vi "Main_Target.vi"() -> ()   [LabVIEW 2018]
uses:
  Tasks_RT.ctl
  ActionCluster.ctl
  Instructions_RT.ctl
  ParameterSubCluster.ctl
panel:
  out "Chart 2":i16(graph)
  out "Chart":u16(graph)
  out "Inbit line":string="6509/port0/line1"
  in  "Action cluster":T1={"Macro Instructions"=[{"Duration (s)"=0.1, "Steps"=1, "Changes"=[FALSE, TRUE, FALSE], "Triggers"=[], "RAW cmds 2D"=[[0, 0, 0, 0, 0, 0, 0, 0], [0, 0, 0, 0, 0, 0, 0, 0], [0, 0, 0, 0, 0, 0, 0, 0], [0, 0, 0, 0, 0, 0, 0, 0], [0, 0, 0, 0, 0, 0, 0, 0], [0, 0, 0, 0, 0, 0, 0, 0], [0, 0, 0, 0, 0, 0, 0, 0], [0, 0, 0, 0, 0, 0, 0, 0], [0, 0, 0, 0, 0, 0, 0, 0], [0, 0, 0, 0, 0, 0, 0, 0], [0, 0, 0, 0, 0, 0, 0, 0], [0, 0, 0, 0, 0, 0, 0, 0], [0, 0, 0, 0, 0, 0, 0, 0], [0, 0, 0, 0, 0, 0, 0, 0], [0, 0, 0, 0, 0, 0, 0, 0], [0, 0, 0, 0, 0, 0, 0, 0], [0, 0, 0, 0, 0, 0, 0, 0], [0, 0, 0, 0, 0, 0, 0, 0], [0, 0, 0, 0, 0, 0, 0, 0], [0, 0, 0, 0, 0, 0, 0, 0], [0, 0, 0, 0, 0, 0, 0, 0], [0, 0, 0, 0, 0, 0, 0, 0], [0, 0, 0, 0, 0, 0, 0, 0], [0, 0, 0, 0, 0, 0, 0, 0], [0, 0, 0, 0, 0, 0, 0, 0], [0, 0, 0, 0, 0, 0, 0, 0], [0, 0, 0, 0, 0, 0, 0, 0], [0, 0, 0, 0, 0, 0, 0, 0], [0, 0, 0, 0, 0, 0, 0, 0], [0, 0, 0, 0, 0, 0, 0, 0], [0, 0, 0, 0, 0, 0, 0, 0], [0, 0, 0, 0, 0, 0, 0, 0], [0, 0, 0, 0, 0, 0, 0, 0], [0, 0, 0, 0, 0, 0, 0, 0], [0, 0, 0, 0, 0, 0, 0, 0], [0, 0, 0, 0, 0, 0, 0, 0], [0, 0, 0, 0, 0, 0, 0, 0], [0, 0, 0, 0, 0, 0, 0, 0], [0, 0, 0, 0, 0, 0, 0, 0], [0, 0, 0, 0, 0, 0, 0, 0], [0, 0, 0, 0, 0, 0, 0, 0], [0, 0, 0, 0, 0, 0, 0, 0], [0, 0, 0, 0, 0, 0, 0, 0], [0, 0, 0, 0, 0, 0, 0, 0], [0, 0, 0, 0, 0, 0, 0, 0], [0, 0, 0, 0, 0, 0, 0, 0], [0, 0, 0, 0, 0, 0, 0, 0], [0, 0, 0, 0, 0, 0, 0, 0], [0, 0, 0, 0, 0, 0, 0, 0], [0, 0, 0, 0, 0, 0, 0, 0], [0, 0, 0, 0, 0, 0, 0, 0], [0, 0, 0, 0, 0, 0, 0, 0], [0, 0, 0, 0, 0, 0, 0, 0], [0, 0, 0, 0, 0, 0, 0, 0], [0, 0, 0, 0, 0, 0, 0, 0], [0, 0, 0, 0, 0, 0, 0, 0], [0, 0, 0, 0, 0, 0, 0, 0], [0, 0, 0, 0, 0, 0, 0, 0], [0, 0, 0, 0, 0, 0, 0, 0], [0, 0, 0, 0, 0, 0, 0, 0], [0, 0, 0, 0, 0, 0, 0, 0], [0, 0, 0, 0, 0, 0, 0, 0], [0, 0, 0, 0, 0, 0, 0, 0], [0, 0, 0, 0, 0, 0, 0, 0], [0, 0, 0, 0, 0, 0, 0, 0], [0, 0, 0, 0, 0, 0, 0, 0], [0, 0, 0, 0, 0, 0, 0, 0], [0, 0, 0, 0, 0, 0, 0, 0], [0, 0, 0, 0, 0, 0, 0, 0], [0, 0, 0, 0, 0, 0, 0, 0], [0, 0, 0, 0, 0, 0, 0, 0], [0, 0, 0, 0, 0, 0, 0, 0], [0, 0, 0, 0, 0, 0, 0, 0], [0, 0, 0, 0, 0, 0, 0, 0], [0, 0, 0, 0, 0, 0, 0, 0], [0, 0, 0, 0, 0, 0, 0, 0], [0, 0, 0, 0, 0, 0, 0, 0], [0, 0, 0, 0, 0, 0, 0, 0], [0, 0, 0, 0, 0, 0, 0, 0], [0, 0, 0, 0, 0, 0, 0, 0], [0, 0, 0, 0, 0, 0, 0, 0], [0, 0, 0, 0, 0, 0, 0, 0], [0, 0, 0, 0, 0, 0, 0, 0], [0, 0, 0, 0, 0, 0, 0, 0], [0, 0, 0, 0, 0, 0, 0, 0], [0, 0, 0, 0, 0, 0, 0, 0], [0, 0, 0, 0, 0, 0, 0, 0], [0, 0, 0, 0, 0, 0, 0, 0], [0, 0, 0, 0, 0, 0, 0, 0], [0, 0, 0, 0, 0, 0, 0, 0], [0, 0, 0, 0, 0, 0, 0, 0], [0, 0, 0, 0, 0, 0, 0, 0], [0, 0, 0, 0, 0, 0, 0, 0], [0, 0, 0, 0, 0, 0, 0, 0], [0, 0, 0, 0, 0, 0, 0, 0], [0, 0, 0, 0, 0, 0, 0, 0], [0, 0, 0, 0, 0, 0, 0, 0], [0, 0, 0, 0, 0, 0, 0, 0], [0, 0, 0, 0, 0, 0, 0, 0], [0, 0, 0, 0, 0, 0, 0, 0], [0, 0, 0, 0, 0, 0, 0, 0], [0, 0, 0, 0, 0, 0, 0, 0], [0, 0, 0, 0, 0, 0, 0, 0], [0, 0, 0, 0, 0, 0, 0, 0], [0, 0, 0, 0, 0, 0, 0, 0], [0, 0, 0, 0, 0, 0, 0, 0], [0, 0, 0, 0, 0, 0, 0, 0], [0, 0, 0, 0, 0, 0, 0, 0], [0, 0, 0, 0, 0, 0, 0, 0], [0, 0, 0, 0, 0, 0, 0, 0], [0, 0, 0, 0, 0, 0, 0, 0], [0, 0, 0, 0, 0, 0, 0, 0], [0, 0, 0, 0, 0, 0, 0, 0], [0, 0, 0, 0, 0, 0, 0, 0], [0, 0, 0, 0, 0, 0, 0, 0], [0, 0, 0, 0, 0, 0, 0, 0], [0, 0, 0, 0, 0, 0, 0, 0], [0, 0, 0, 0, 0, 0, 0, 0], [0, 0, 0, 0, 0, 0, 0, 0], [0, 0, 0, 0, 0, 0, 0, 0], [0, 0, 0, 0, 0, 0, 0, 0], [0, 0, 0, 0, 0, 0, 0, 0], [0, 0, 0, 0, 0, 0, 0, 0], [0, 0, 0, 0, 0, 0, 0, 0], [0, 0, 0, 0, 0, 0, 0, 0], [0, 0, 0, 0, 0, 0, 0, 0], [0, 0, 0, 0, 0, 0, 0, 0], [0, 0, 0, 0, 0, 0, 0, 0], [0, 0, 0, 0, 0, 0, 0, 0], [0, 0, 0, 0, 0, 0, 0, 0], [0, 0, 0, 0, 0, 0, 0, 0], [0, 0, 0, 0, 0, 0, 0, 0], [0, 0, 0, 0, 0, 0, 0, 0], [0, 0, 0, 0, 0, 0, 0, 0], [0, 0, 0, 0, 0, 0, 0, 0], [0, 0, 0, 0, 0, 0, 0, 0], [0, 0, 0, 0, 0, 0, 0, 0], [0, 0, 0, 0, 0, 0, 0, 0], [0, 0, 0, 0, 0, 0, 0, 0], [0, 0, 0, 0, 0, 0, 0, 0], [0, 0, 0, 0, 0, 0, 0, 0], [0, 0, 0, 0, 0, 0, 0, 0], [0, 0, 0, 0, 0, 0, 0, 0], [0, 0, 0, 0, 0, 0, 0, 0], [0, 0, 0, 0, 0, 0, 0, 0], [0, 0, 0, 0, 0, 0, 0, 0], [0, 0, 0, 0, 0, 0, 0, 0], [0, 0, 0, 0, 0, 0, 0, 0], [0, 0, 0, 0, 0, 0, 0, 0], [0, 0, 0, 0, 0, 0, 0, 0], [0, 0, 0, 0, 0, 0, 0, 0], [0, 0, 0, 0, 0, 0, 0, 0], [0, 0, 0, 0, 0, 0, 0, 0], [0, 0, 0, 0, 0, 0, 0, 0], [0, 0, 0, 0, 0, 0, 0, 0], [0, 0, 0, 0, 0, 0, 0, 0], [0, 0, 0, 0, 0, 0, 0, 0], [0, 0, 0, 0, 0, 0, 0, 0], [0, 0, 0, 0, 0, 0, 0, 0], [0, 0, 0, 0, 0, 0, 0, 0], [0, 0, 0, 0, 0, 0, 0, 0], [0, 0, 0, 0, 0, 0, 0, 0], [0, 0, 0, 0, 0, 0, 0, 0], [0, 0, 0, 0, 0, 0, 0, 0], [0, 0, 0, 0, 0, 0, 0, 0], [0, 0, 0, 0, 0, 0, 0, 0], [0, 0, 0, 0, 0, 0, 0, 0], [0, 0, 0, 0, 0, 0, 0, 0], [0, 0, 0, 0, 0, 0, 0, 0], [0, 0, 0, 0, 0, 0, 0, 0], [0, 0, 0, 0, 0, 0, 0, 0], [0, 0, 0, 0, 0, 0, 0, 0], [0, 0, 0, 0, 0, 0, 0, 0], [0, 0, 0, 0, 0, 0, 0, 0], [0, 0, 0, 0, 0, 0, 0, 0], [0, 0, 0, 0, 0, 0, 0, 0], [0, 0, 0, 0, 0, 0, 0, 0], [0, 0, 0, 0, 0, 0, 0, 0], [0, 0, 0, 0, 0, 0, 0, 0], [0, 0, 0, 0, 0, 0, 0, 0], [0, 0, 0, 0, 0, 0, 0, 0], [0, 0, 0, 0, 0, 0, 0, 0], [0, 0, 0, 0, 0, 0, 0, 0], [0, 0, 0, 0, 0, 0, 0, 0], [0, 0, 0, 0, 0, 0, 0, 0], [0, 0, 0, 0, 0, 0, 0, 0], [0, 0, 0, 0, 0, 0, 0, 0], [0, 0, 0, 0, 0, 0, 0, 0], [0, 0, 0, 0, 0, 0, 0, 0], [0, 0, 0, 0, 0, 0, 0, 0], [0, 0, 0, 0, 0, 0, 0, 0], [0, 0, 0, 0, 0, 0, 0, 0], [0, 0, 0, 0, 0, 0, 0, 0], [0, 0, 0, 0, 0, 0, 0, 0], [0, 0, 0, 0, 0, 0, 0, 0], [0, 0, 0, 0, 0, 0, 0, 0], [0, 0, 0, 0, 0, 0, 0, 0], [0, 0, 0, 0, 0, 0, 0, 0], [0, 0, 0, 0, 0, 0, 0, 0], [0, 0, 0, 0, 0, 0, 0, 0], [0, 0, 0, 0, 0, 0, 0, 0], [0, 0, 0, 0, 0, 0, 0, 0], [0, 0, 0, 0, 0, 0, 0, 0], [0, 0, 0, 0, 0, 0, 0, 0], [0, 0, 0, 0, 0, 0, 0, 0], [0, 0, 0, 0, 0, 0, 0, 0], [0, 0, 0, 0, 0, 0, 0, 0], [0, 0, 0, 0, 0, 0, 0, 0], [0, 0, 0, 0, 0, 0, 0, 0], [0, 0, 0, 0, 0, 0, 0, 0], [0, 0, 0, 0, 0, 0, 0, 0], [0, 0, 0, 0, 0, 0, 0, 0], [0, 0, 0, 0, 0, 0, 0, 0], [0, 0, 0, 0, 0, 0, 0, 0], [0, 0, 0, 0, 0, 0, 0, 0], [0, 0, 0, 0, 0, 0, 0, 0], [0, 0, 0, 0, 0, 0, 0, 0], [0, 0, 0, 0, 0, 0, 0, 0], [0, 0, 0, 0, 0, 0, 0, 0], [0, 0, 0, 0, 0, 0, 0, 0], [0, 0, 0, 0, 0, 0, 0, 0], [0, 0, 0, 0, 0, 0, 0, 0], [0, 0, 0, 0, 0, 0, 0, 0], [0, 0, 0, 0, 0, 0, 0, 0], [0, 0, 0, 0, 0, 0, 0, 0], [0, 0, 0, 0, 0, 0, 0, 0], [0, 0, 0, 0, 0, 0, 0, 0], [0, 0, 0, 0, 0, 0, 0, 0], [0, 0, 0, 0, 0, 0, 0, 0], [0, 0, 0, 0, 0, 0, 0, 0], [0, 0, 0, 0, 0, 0, 0, 0], [0, 0, 0, 0, 0, 0, 0, 0], [0, 0, 0, 0, 0, 0, 0, 0], [0, 0, 0, 0, 0, 0, 0, 0], [0, 0, 0, 0, 0, 0, 0, 0], [0, 0, 0, 0, 0, 0, 0, 0], [0, 0, 0, 0, 0, 0, 0, 0], [0, 0, 0, 0, 0, 0, 0, 0], [0, 0, 0, 0, 0, 0, 0, 0], [0, 0, 0, 0, 0, 0, 0, 0], [0, 0, 0, 0, 0, 0, 0, 0], [0, 0, 0, 0, 0, 0, 0, 0], [0, 0, 0, 0, 0, 0, 0, 0], [0, 0, 0, 0, 0, 0, 0, 0], [0, 0, 0, 0, 0, 0, 0, 0], [0, 0, 0, 0, 0, 0, 0, 0], [0, 0, 0, 0, 0, 0, 0, 0], [0, 0, 0, 0, 0, 0, 0, 0], [0, 0, 0, 0, 0, 0, 0, 0], [0, 0, 0, 0, 0, 0, 0, 0], [0, 0, 0, 0, 0, 0, 0, 0], [0, 0, 0, 0, 0, 0, 0, 0], [0, 0, 0, 0, 0, 0, 0, 0], [0, 0, 0, 0, 0, 0, 0, 0], [0, 0, 0, 0, 0, 0, 0, 0]]}], "Slow AO Array"=[{"ao line"="ao0", "Initial, Final"=[0.0, 0.0]}, {"ao line"="ao1", "Initial, Final"=[0.0, 0.0]}, {"ao line"="ao14", "Initial, Final"=[0.0, 0.0]}], "Duration (s)"=0.1}
  in  "PXI card names":string[](array[string])=["DIO:", "6509", "Counter:", "6733_1", "Fast AO:", "6733_1", "6733_2", "Slow AO:", "6723"]
  out "Task cluster":T4={"Outbits"="Outbits", "Counter"="Counter", "Digital Input Device"="6509", "Slow AO Device"="6723", "Fast AO"=["Fast AO_1", "Fast AO_2"], "Error Array"=[{"status"=FALSE, "code"=0, "source"=""}, {"status"=FALSE, "code"=0, "source"=""}, {"status"=FALSE, "code"=0, "source"=""}, {"status"=FALSE, "code"=0, "source"=""}], "outbits"=38, "inbits"=8}
  in  "Min Loop Time (us)":u32=10000
  in  "stop":bool
  # "Tasks and errors"
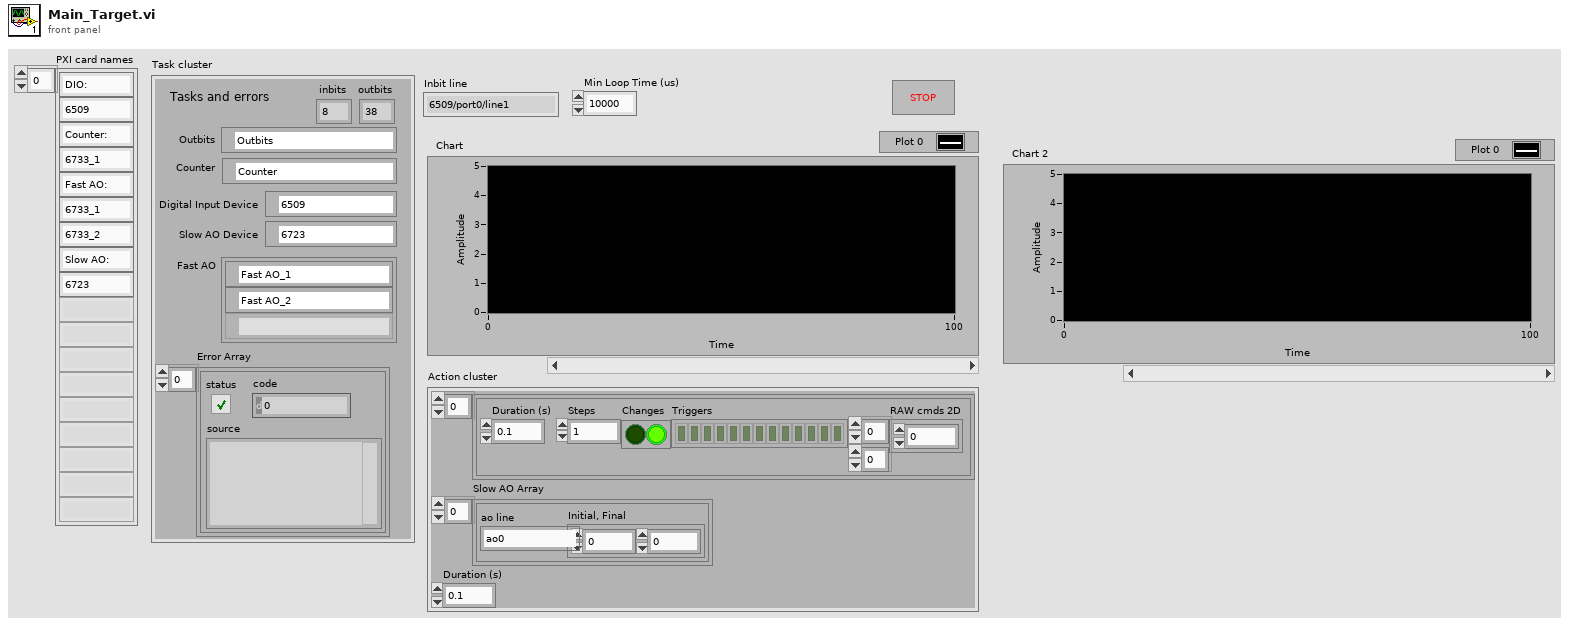
[diagram p1: front panel]
types:
  T1 = typedef "ActionCluster.ctl" = cluster{"Macro Instructions":T2, "Slow AO Array":T3, "Duration (s)":dbl}
  T2 = typedef "Instructions_RT.ctl" = cluster{"Duration (s)":dbl, "Steps":i32, "Changes":bool[], "Triggers":bool[], "RAW cmds 2D":i16[][]}[]
  T3 = typedef "ParameterSubCluster.ctl" = cluster{"ao line":string, "Initial, Final":dbl[]}[]
  T4 = typedef "Tasks_RT.ctl" = cluster{"Outbits":refnum<k21>, "Counter":refnum<k21>, "Digital Input Device":tag, "Slow AO Device":tag, "Fast AO":refnum<k21>[], "Error Array":errorcluster[], "outbits":i32, "inbits":i32}
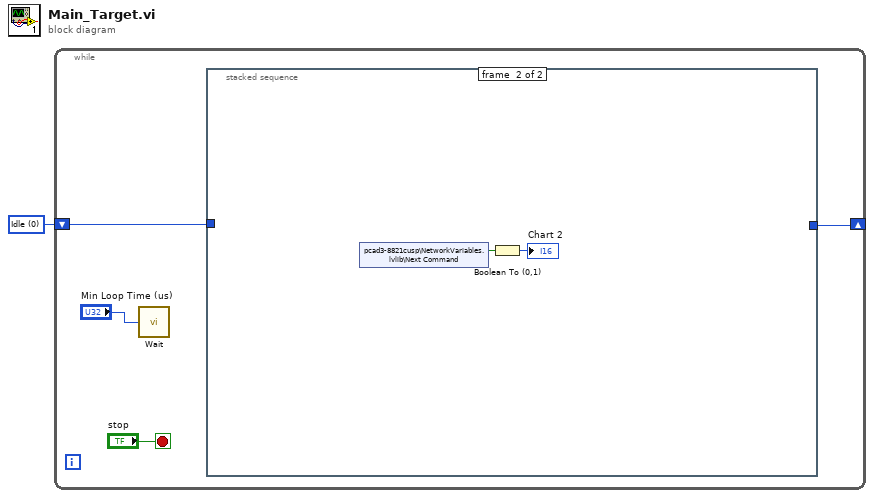
[diagram p0: block diagram]
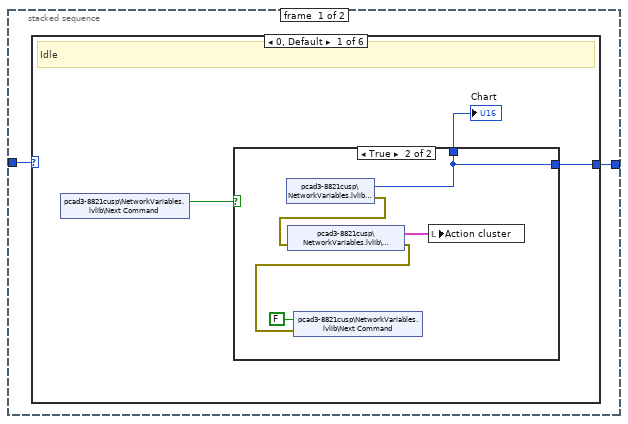
[diagram p2: hidden frame]
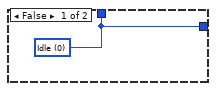
[diagram p3: hidden frame]
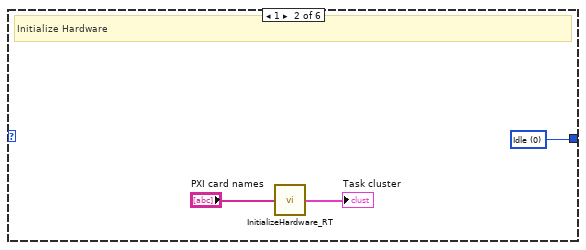
[diagram p4: hidden frame]
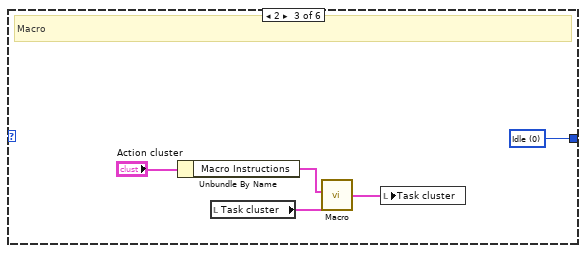
[diagram p5: hidden frame]
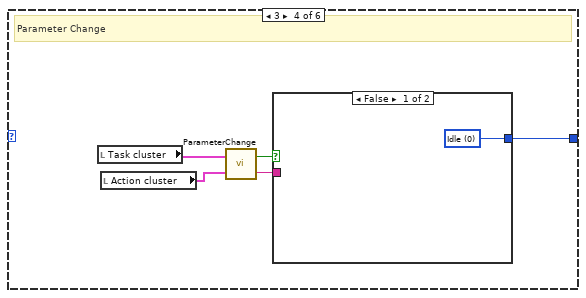
[diagram p6: hidden frame]
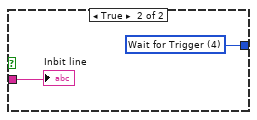
[diagram p7: hidden frame]
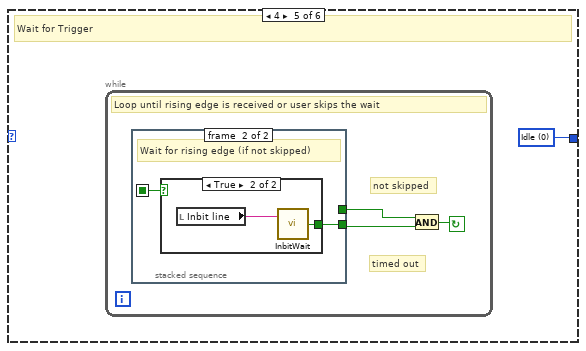
[diagram p8: hidden frame]
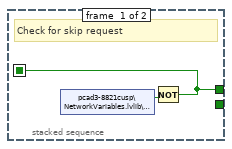
[diagram p9: hidden frame]
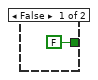
[diagram p10: hidden frame]
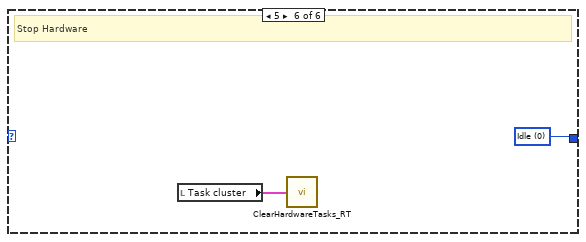
[diagram p11: hidden frame]
diagram:
  w1 = u16 0 items=["Idle", "Initialize Hardware", "Macro", "Parameter Change", "Wait for Trigger", "Stop Hardware"] ("State")
  n1 = while {
    shift-right: [w3] -> _
    shift-left: w1 -> [w2]
    stop <- "stop" stop-if-true
    n2 = call "Wait"("Count(uSec)"="Min Loop Time (us)") -> ()  [unwired: 1 out]
    n3 = stacked-sequence {
      tunnel: [w7 _] -> w3
      tunnel: w2 -> [w6 _]
      frame #0 {
        n4 = case shown="0, Default" w6 {
          tunnel: [w8 w17 w20 w25 w33 w45] -> w7
          frame 0, Default {
            # "Idle"
            n5 = shared-variable "pcad3-8821cusp\\NetworkVariables.lvlib\\Next Command"() -> (w9:bool)  [unwired: 1 in, 1 out]
            n6 = case shown="True" w9 {
              tunnel: [w11 w12] -> w10
              tunnel: [w11 w12] -> w8
              frame False {
                w11 = u16 0 items=["Idle", "Initialize Hardware", "Macro", "Parameter Change", "Wait for Trigger", "Stop Hardware"] ("State")
              }
              frame True {
                n7 = shared-variable "pcad3-8821cusp\\NetworkVariables.lvlib\\RT State"() -> (w12:u16, error out=w15:errorcluster)  [unwired: 1 in]
                n8 = shared-variable "pcad3-8821cusp\\NetworkVariables.lvlib\\ActionCluster"(error in=w15) -> (w16:T1, error out=w13:errorcluster)
                n9 = shared-variable "pcad3-8821cusp\\NetworkVariables.lvlib\\Next Command"(FALSE ("Next Command"), error in=w13) -> ()  [unwired: 1 out]
                n10 = local write "Action cluster"(w16) -> ()
              }
            }
            "Chart" <- w10
          }
          frame 1 {
            w17 = u16 0 items=["Idle", "Initialize Hardware", "Macro", "Parameter Change", "Wait for Trigger", "Stop Hardware"] ("State")
            # "Initialize Hardware"
            n11 = call "InitializeHardware_RT.vi"("PXI card names"="PXI card names") -> ("Task cluster"=→"Task cluster":T4)
          }
          frame 2 {
            w20 = u16 0 items=["Idle", "Initialize Hardware", "Macro", "Parameter Change", "Wait for Trigger", "Stop Hardware"] ("State")
            # "Macro"
            n12 = Unbundle By Name("Action cluster") -> ("Macro Instructions"=w23:T2)
            n13 = local read "Task cluster"() -> (w21:T4)
            n14 = call "Macro.vi"("Macro Instructions"=w23, "Tasks in"=w21) -> ("Tasks out"=w22:T4)  [unwired: 3 in]
            n15 = local write "Task cluster"(w22) -> ()
          }
          frame 3 {
            # "Parameter Change"
            n16 = local read "Task cluster"() -> (w29:T4)
            n17 = local read "Action cluster"() -> (w28:T1)
            n18 = call "ParameterChange.vi"("Action"=w28, "Tasks in"=w29) -> ("inbit line"=w26:string, "Wait for inbit"=w27:bool)
            n19 = case shown="False" w27 {
              tunnel: w26 -> [_ w32]
              tunnel: [w30 w31] -> w25
              frame False {
                w30 = u16 0 items=["Idle", "Initialize Hardware", "Macro", "Parameter Change", "Wait for Trigger", "Stop Hardware"] ("State")
              }
              frame True {
                w31 = u16 4 items=["Idle", "Initialize Hardware", "Macro", "Parameter Change", "Wait for Trigger", "Stop Hardware"] ("State")
                "Inbit line" <- w32
              }
            }
          }
          frame 4 {
            w33 = u16 0 items=["Idle", "Initialize Hardware", "Macro", "Parameter Change", "Wait for Trigger", "Stop Hardware"] ("State")
            # "Wait for Trigger"
            n20 = while {
              stop <- w36 continue-if-true
              # "timed out"
              # "not skipped"
              # "Loop until rising edge is received or user skips the wait"
              n21 = stacked-sequence {
                seq-local: [w37 _] -> [_ w39]
                tunnel: [_ w40] -> w35
                tunnel: [w37 _] -> w34
                frame #0 {
                  # "Check for skip request"
                  n22 = shared-variable "pcad3-8821cusp\\NetworkVariables.lvlib\\Skip Wait"() -> (w38:bool)  [unwired: 1 in, 1 out]
                  n23 = Not(x=w38) -> (.not. x?=w37:bool)
                }
                frame #1 {
                  # "Wait for rising edge (if not skipped)"
                  n24 = case shown="True" w39 {
                    tunnel: [FALSE ("Timed out") w42] -> w40
                    frame False {
                    }
                    frame True {
                      n25 = local read "Inbit line"() -> (w43:string)
                      n26 = call "InbitWait.vi"("Inbit line"=w43) -> ("Timed out"=w42:bool)  [unwired: 1 in]
                    }
                  }
                }
              }
              n27 = And(x=w34, y=w35) -> (x .and. y?=w36:bool)
            }
          }
          frame 5 {
            w45 = u16 0 items=["Idle", "Initialize Hardware", "Macro", "Parameter Change", "Wait for Trigger", "Stop Hardware"] ("State")
            # "Stop Hardware"
            n28 = local read "Task cluster"() -> (w44:T4)
            n29 = call "ClearHardwareTasks_RT.vi"("Task cluster"=w44) -> ()  [unwired: 1 in]
          }
        }
      }
      frame #1 {
        n30 = shared-variable "pcad3-8821cusp\\NetworkVariables.lvlib\\Next Command"() -> (w47:bool)  [unwired: 1 in, 1 out]
        n31 = Boolean To (0,1)(Boolean=w47) -> (0, 1=→"Chart 2":i16)
      }
    }
  }
